vi "value log.vi"() -> ()   [LabVIEW 2013]
panel:
  out "time":string
  in  "Path":path=path "C:/Snap-On_GEP_M2/trunk/Software/Test Sequence/Value log.txt"
  in  "Value":dbl
  in  "Serial Number":string
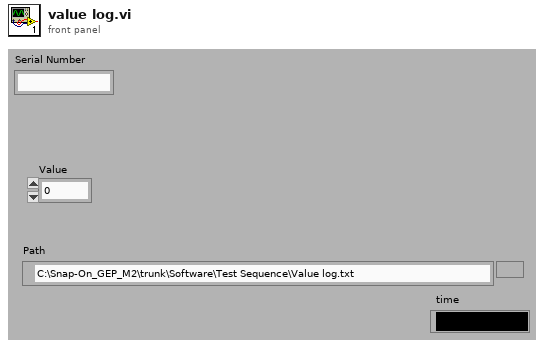
[diagram p1: front panel]
types:
  T1 = enum16{"open", "replace", "create", "open or create", "replace or create", "replace or create with confirmation"}
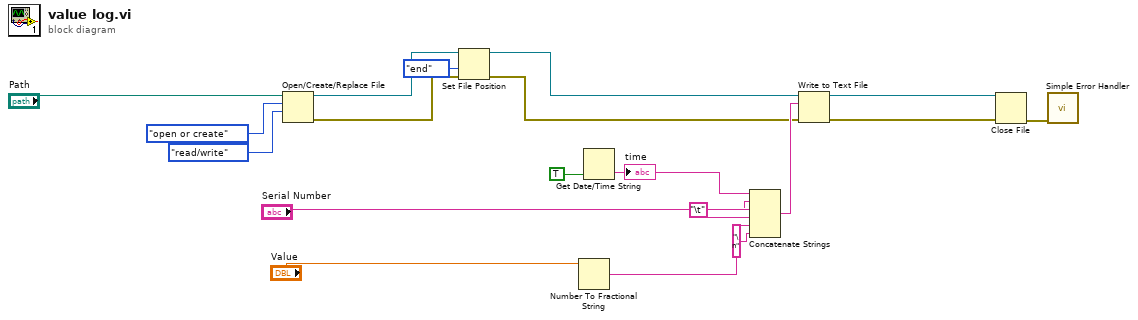
[diagram p0: block diagram]
diagram:
  w10 = "\t" ("Tab")
  n1 = Open/Create/Replace File(file path (use dialog)="Path", operation (0:open)=T1."open or create", access (0:read/write)=enum16{"read/write", "read-only", "write-only"}."read/write") -> (refnum out=w4:refnum<file>, error out=w5:errorcluster)  [unwired: 3 in, 1 out]
  n2 = Set File Position(refnum=w4, from (0:start)=enum16{"start", "end", "current"}."end", error in=w5) -> (refnum out=w3:refnum<file>, error out=w2:errorcluster)  [unwired: 1 in]
  n3 = Number To Fractional String(number="Value") -> (F-format string=w8:string)  [unwired: 3 in]
  n4 = Get Date/Time String(want seconds? (F)=TRUE) -> (time string=w12:string)  [unwired: 2 in, 1 out]
  "time" <- w12
  n5 = Concatenate Strings(w12, w10, "Serial Number", w10, w8, "\n" ("string")) -> (w14:string)
  n6 = Write to Text File(file (use dialog)=w3, text=w14, error in=w2) -> (refnum out=w19:refnum<file>, error out=w18:errorcluster)  [unwired: 1 in, 1 out]
  n7 = Close File(refnum=w19, error in=w18) -> (error out=w17:errorcluster)  [unwired: 1 out]
  n8 = call <vilib>:"Simple Error Handler.vi"("error in (no error)"=w17) -> ()  [unwired: 4 in, 5 out]
